vi "Module 1 Cases.vi"() -> ()   [LabVIEW 2024]
uses:
  Module 1 Cases.ctl
  Channel Messages/Sum.ctl
panel:
  out "Module 1 Cases":map{T1, variant}(c390)
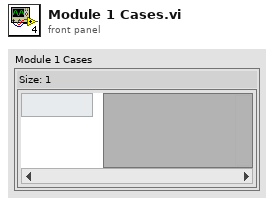
[diagram p1: front panel]
types:
  T1 = typedef "Module 1 Cases.ctl" = enum16{"Kill", "Stop", "Init", "Sum"}
  T2 = typedef "Sum.ctl" = cluster{"summand0":dbl, "summand1":dbl}
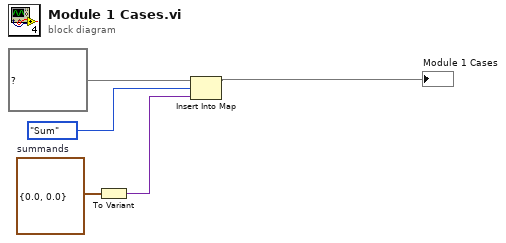
[diagram p0: block diagram]
diagram:
  w3 = T2 {"summand0"=0.0, "summand1"=0.0}  # summands
  n1 = To Variant(anything=w3) -> (Variant=w2:variant)
  n2 = Insert Into Map(map in=map{T1, variant} {}, key=Module_1_Cases."Sum", value=w2) -> (map out=→"Module 1 Cases":map{T1, variant})  [unwired: 2 out]
